vi "Global Correct Answer.vi"() -> ()   [LabVIEW 2020]
panel:
  in  "CorrectAnswer":bool
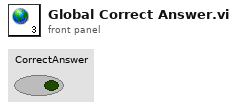
[diagram p1: front panel]
diagram:
